vi "RG Configure DAQ auto Max input scale.vi"(4 "input terminal configuration":i32(ring)=10106 items=["default"=-1, "RSE"=10083, "NRSE"=10078, "Differential"=10106, "Pseudodifferential"=12529], 6 "DAQ Card Type":enum16{"USB-6211", "USB-6251"}(ring), 7 "Sampling rate":dbl=20000.0, 8 "error in":errorcluster, 9 "DAQ Trigger Level":dbl format="%0.2f", 10 "physical channel":string="Dev2/ai0", 11 "number of samples":i32=100000) -> (0 "error out":errorcluster, 3 "task out":refnum<k21>)   [LabVIEW 2015]
uses:
  <vilib>/DAQmx/read.llb/DAQmx Read (Analog Wfm 1Chan NSamp).vi
  <vilib>/Analysis/baseanly.llb/Mean (DBL).vi
  <vilib>/DAQmx/configure/trigger.llb/DAQmx Trigger.vi
  <vilib>/DAQmx/configure/trigger.llb/DAQmx Reference Trigger (Analog Edge).vi
  <vilib>/DAQmx/configure/trigger.llb/DAQmx Reference Trigger (Digital Edge).vi
  <vilib>/DAQmx/configure/timing.llb/DAQmx Timing (Sample Clock).vi
  <vilib>/DAQmx/miscellaneous.llb/DAQmx Fill In Error Info.vi
  <vilib>/DAQmx/create/channels.llb/DAQmx Create Channel (AI-Voltage-Basic).vi
  <vilib>/Analysis/NI_AALBase.lvlib
  <resource>/objmgr/daqmx.rc
panel:
  out "Input Maximum":dbl format="%#_13g"
  out "pre-trigger samples":u32=10000
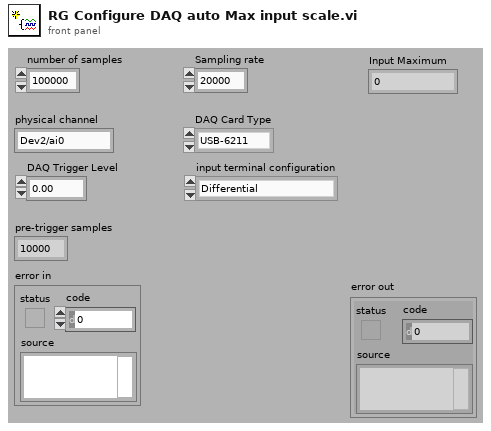
[diagram p1: front panel]
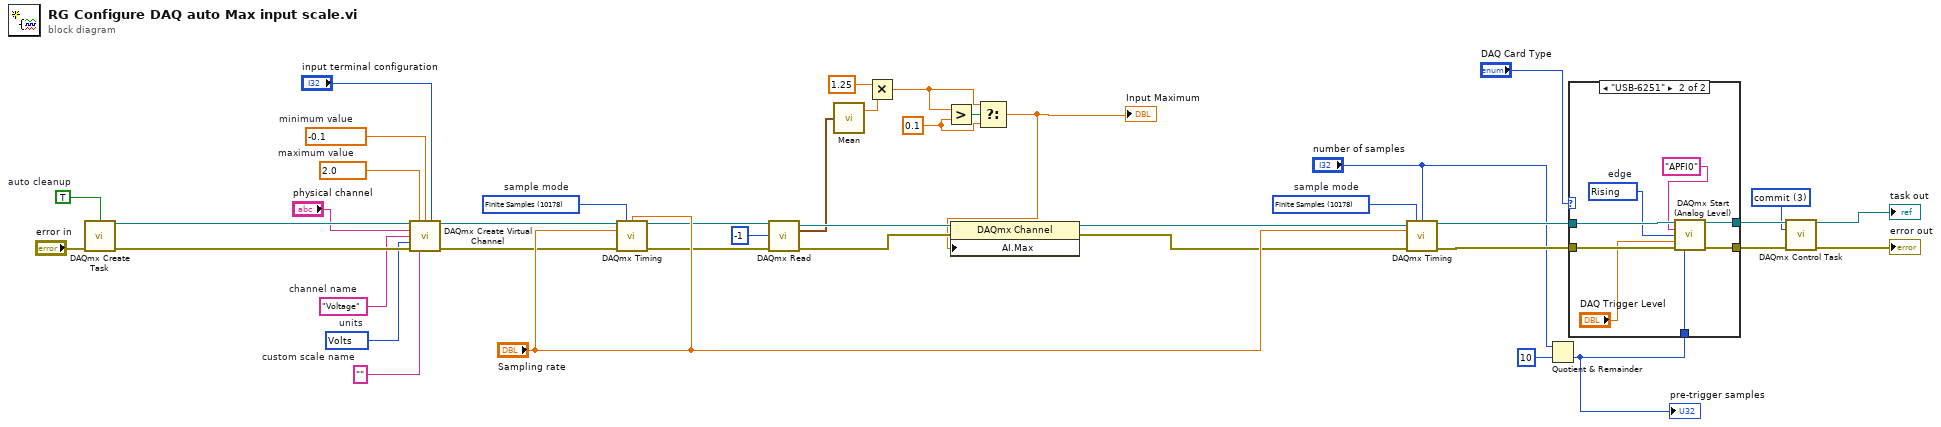
[diagram p0: block diagram]
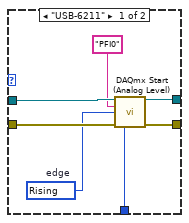
[diagram p2: hidden frame]
diagram:
  w9 = 0.1 ("y")
  w23 = 10178 items=["Finite Samples"=10178, "Continuous Samples"=10123, "Hardware Timed Single Point"=12522]  # sample mode
  w24 = 3 items=["verify"=2, "reserve"=4, "commit"=3, "unreserve"=5, "abort"=6] ("action")
  w34 = 10178 items=["Finite Samples"=10178, "Continuous Samples"=10123, "Hardware Timed Single Point"=12522]  # sample mode
  w14 = 10348 items=["Volts"=10348, "From Custom Scale"=10065]  # units
  w13 = "Voltage"  # channel name
  w36 = ""  # custom scale name
  w12 = -0.1  # minimum value
  w37 = 2.0  # maximum value
  w39 = TRUE  # auto cleanup
  n1 = call <vilib>:"DAQmx Create Task.vi"("auto cleanup"=w39, "error in"="error in") -> ("task out"=w38:refnum<k21>, "error out"=w40:errorcluster)  [unwired: 12 in]
  n2 = call-poly <vilib>:"DAQmx Create Virtual Channel.vi"("task in"=w38, "maximum value"=w37, "minimum value"=w12, "input terminal configuration"="input terminal configuration", "physical channels"="physical channel", "name to assign"=w13, "units"=w14, "error in"=w40, "custom scale name"=w36) -> ("task out"=w20:refnum<k21>, "error out"=w21:errorcluster)  [unwired: 5 in]
  n3 = call-poly <vilib>:"DAQmx Timing.vi"("task/channels in"=w20, "sample mode"=w23, "samples per channel"="Sampling rate", "rate"="Sampling rate", "error in"=w21) -> ("task out"=w19:refnum<k21>, "error out"=w18:errorcluster)  [unwired: 9 in]
  n4 = call-poly <vilib>:"DAQmx Read.vi"("task/channels in"=w19, "number of samples per channel"=-1, "error in"=w18) -> ("task out"=w6:refnum<k21>, "data"=w1:waveform(dbl), "error out"=w5:errorcluster)  [unwired: 10 in]
  n5 = call-poly <vilib>:"Mean.vi"("X"=w1) -> ("mean"=w17:dbl)  [unwired: 1 out]
  n6 = Multiply(x=1.25, y=w17) -> (x*y=w8:dbl)
  n7 = Greater?(x=w8, y=w9) -> (0:w10:bool)
  n8 = Select(t=w8, s=w10, f=w9) -> (s? t:f=w4:dbl)
  "Input Maximum" <- w4
  n9 = property class="DAQmx Channel"(reference=w6, error in=w5, "AI.Max"=w4) -> (reference out=w3:refnum<k21>, error out=w2:errorcluster)
  n10 = call-poly <vilib>:"DAQmx Timing.vi"("task/channels in"=w3, "sample mode"=w34, "samples per channel"="number of samples", "rate"="Sampling rate", "error in"=w2) -> ("task out"=w33:refnum<k21>, "error out"=w35:errorcluster)  [unwired: 9 in]
  n11 = Quotient & Remainder(x="number of samples", y=10) -> (floor(x/y)=w30:i32)  [unwired: 1 out]
  "pre-trigger samples" <- w30
  n12 = case shown="\"USB-6251\"" "DAQ Card Type" {
    tunnel: w35 -> [w48 w56]
    tunnel: [w47 w55] -> w28
    tunnel: [w46 w54] -> w27
    tunnel: w33 -> [w45 w53]
    tunnel: w30 -> [w42 w50]
    frame "USB-6211" {
      w44 = 10280 items=["Rising"=10280, "Falling"=10171]  # edge
      n13 = call-poly "DAQmx Start (Analog Level).vi"("task/channels in"=w45, "source"="PFI0", "edge"=w44, "error in"=w48, "pretrigger samples per channel"=w42) -> ("task out"=w47:refnum<k21>, "error out"=w46:errorcluster)  [unwired: 9 in]
    }
    frame "USB-6251" {
      w52 = 10280 items=["Rising"=10280, "Falling"=10171]  # edge
      n14 = call-poly "DAQmx Start (Analog Level).vi"("task/channels in"=w53, "source"="APFI0", "slope"=w52, "level"="DAQ Trigger Level", "error in"=w56, "pretrigger samples per channel"=w50) -> ("task out"=w55:refnum<k21>, "error out"=w54:errorcluster)  [unwired: 8 in]
    }
  }
  n15 = call <vilib>:"DAQmx Control Task.vi"("task/channels in"=w28, "action"=w24, "error in"=w27) -> ("task out"=→"task out":refnum<k21>, "error out"=→"error out":errorcluster)  [unwired: 11 in]
